vi "InitStubs.vi"   [LabVIEW 2013]
uses:
  ValvesValuesStub.vi
  MeasureStateStub.vi
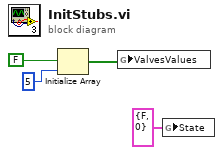
[diagram p0: block diagram]
diagram:
  n1 = Initialize Array(FALSE, 5) -> (w4:bool[])
  n2 = global write "ValvesValuesStub.vi" "ValvesValues"(w4) -> ()
  n3 = global write "MeasureStateStub.vi" "State"(cluster{bool, "CalibrationState":u32} {FALSE, "CalibrationState"=0} ("State")) -> ()
